vi "arrayrevise.vi"(10 "in":bool[](array[boolean])) -> (2 "out":bool[](array[boolean]))   [LabVIEW 2012]
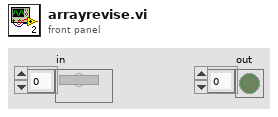
[diagram p1: front panel]
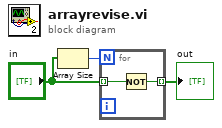
[diagram p0: block diagram]
diagram:
  n1 = Array Size(array="in") -> (size(s)=w3:i32)
  n2 = for {
    N: w3 -> [_]
    tunnel: "in" -> [w5] mode=indexing
    tunnel: [w4] -> w1 mode=indexing
    n3 = Not(x=w5) -> (.not. x?=w4:bool)
  }
  "out" <- w1
